vi "Init GU Arrange.vi"(6 "Force Auto(False)":bool, 8 "error in":errorcluster, 9 "Latest Cal Cfg":T1, 10 "Curr Cal Cfg In":T1, 11 "Config Data":T2(array[cluster])) -> (0 "error out":errorcluster, 2 "Curr Cal Cfg Out":T1, 3 "Config Data Out":T2(array[cluster]))   [LabVIEW 2020, in "GUCalibration2.lvlib"]
uses:
  GUCalibration2.lvlib
  Controls/Config Data Type.ctl
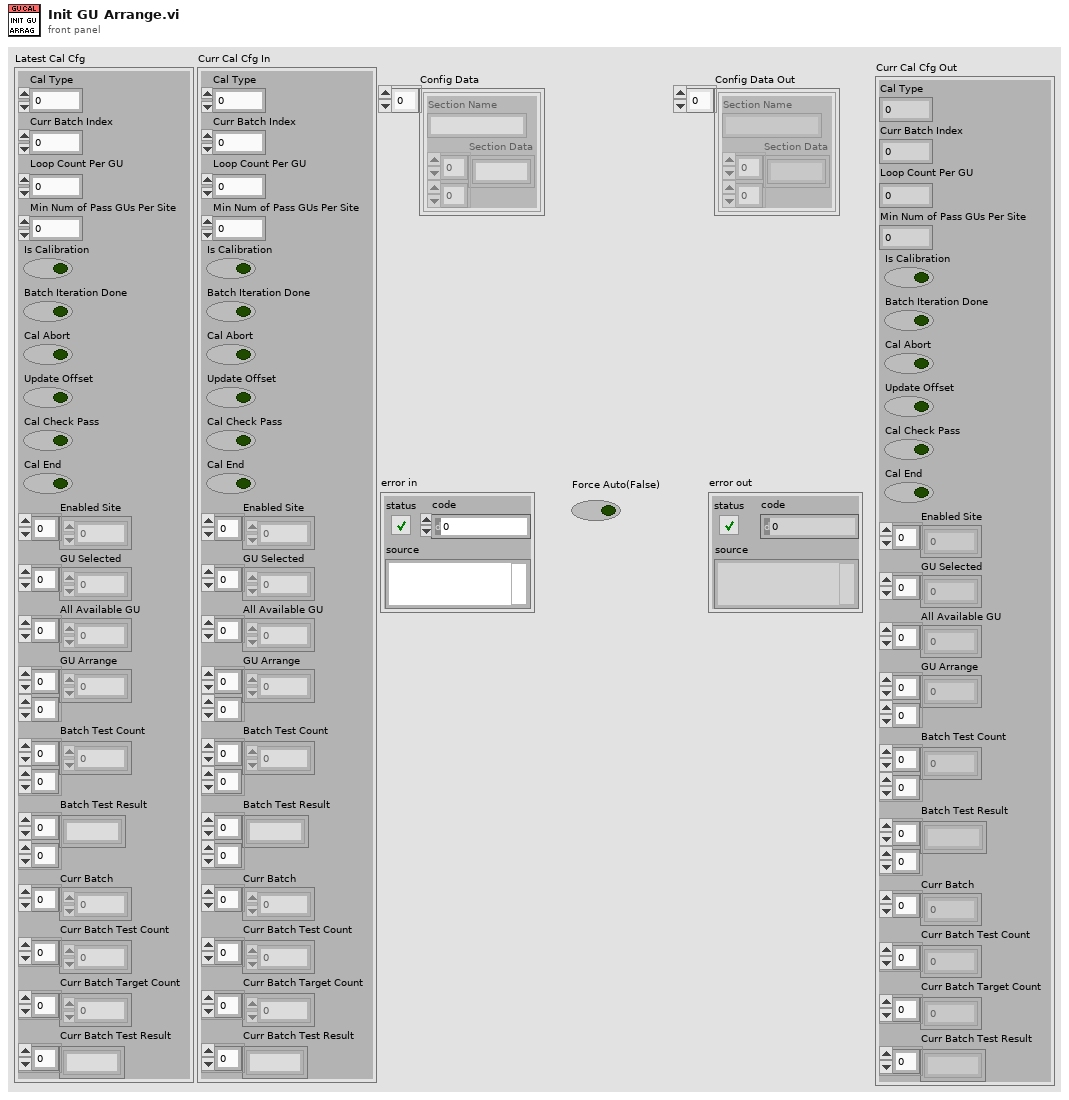
[diagram p1: front panel]
types:
  T1 = typedef "GUCalibration2.lvlib/Config Data Type.ctl" = cluster{"Cal Type":i32, "Curr Batch Index":i32, "Loop Count Per GU":i32, "Min Num of Pass GUs Per Site":i32, "Is Calibration":bool, "Batch Iteration Done":bool, "Cal Abort":bool, "Update Offset":bool, "Cal Check Pass":bool, "Cal End":bool, "Enabled Site":i32[], "GU Selected":i32[], "All Available GU":i32[], "GU Arrange":i32[][], "Batch Test Count":i32[][], "Batch Test Result":string[][], "Curr Batch":i32[], "Curr Batch Test Count":i32[], "Curr Batch Target Count":i32[], "Curr Batch Test Result":string[]}
  T2 = cluster{"Section Name":string, "Section Data":string[][]}[]
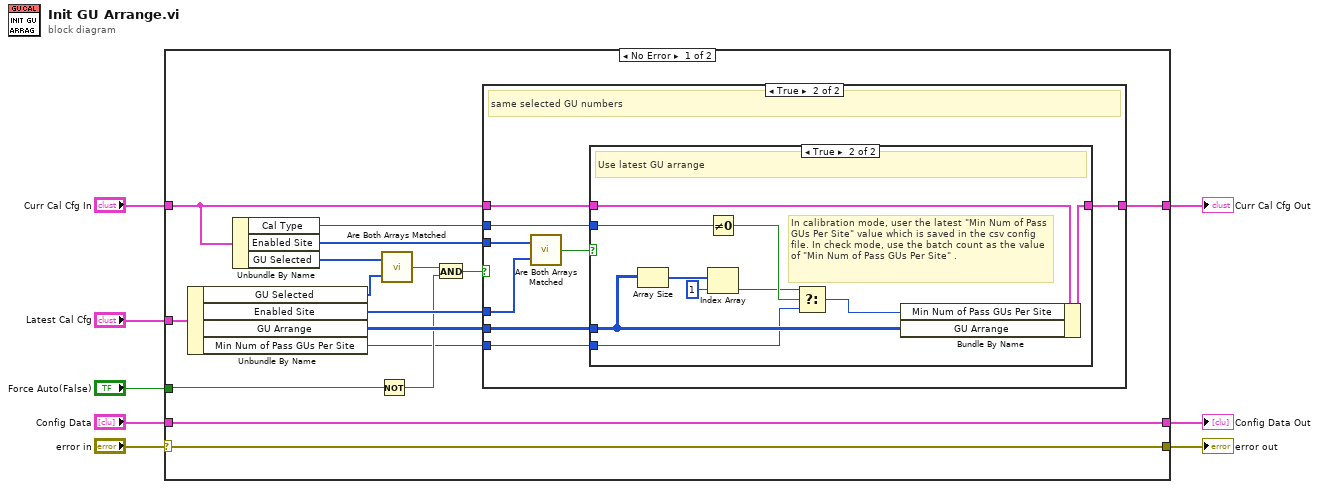
[diagram p0: block diagram]
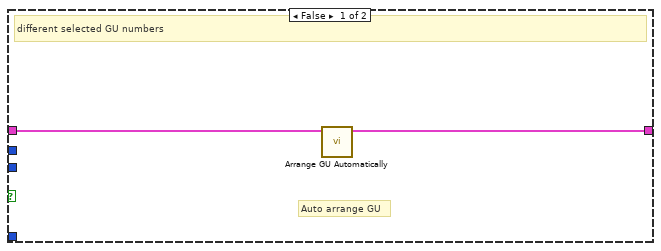
[diagram p2: hidden frame]
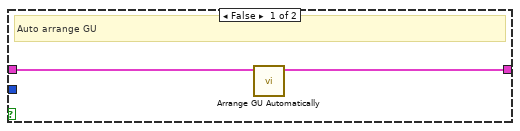
[diagram p3: hidden frame]
diagram:
  n1 = case shown="No Error" "error in" {
    selector: "error in" -> [w16 w49]
    tunnel: [w16 w49] -> w8
    tunnel: "Latest Cal Cfg" -> [w24 _]
    tunnel: "Config Data" -> [w17 w48]
    tunnel: [w17 w48] -> w4
    tunnel: "Curr Cal Cfg In" -> [w19 w47]
    tunnel: [w18 w47] -> w2
    tunnel: "Force Auto(False)" -> [w14 _]
    frame No Error {
      n2 = Unbundle By Name(w24) -> ("GU Selected"=w15:i32[], "Enabled Site"=w22:i32[], "GU Arrange"=w20:i32[][], "Min Num of Pass GUs Per Site"=w10:i32)
      n3 = Unbundle By Name(w19) -> ("Cal Type"=w9:i32, "Enabled Site"=w23:i32[], "GU Selected"=w21:i32[])
      n4 = Not(x=w14) -> (.not. x?=w12:bool)
      n5 = call "Are Both Arrays Matched.vi"("Array2"=w15, "Array1"=w21) -> ("Match ?"=w13:bool)
      n6 = And(x=w13, y=w12) -> (x .and. y?=w11:bool)
      n7 = case shown="True" w11 {
        tunnel: w23 -> [_ w34]
        tunnel: w22 -> [_ w33]
        tunnel: w20 -> [_ w31]
        tunnel: w19 -> [w26 w32]
        tunnel: [w25 w29] -> w18
        tunnel: w10 -> [_ w28]
        tunnel: w9 -> [_ w27]
        frame False {
          # "Auto arrange GU"
          # "different selected GU numbers"
          n8 = call "Arrange GU Automatically.vi"("Curr Cal Cfg In"=w26) -> ("Curr Cal Cfg Out"=w25:T1)  [unwired: 9 in, 1 out]
        }
        frame True {
          # "same selected GU numbers"
          n9 = call "Are Both Arrays Matched.vi"("Array2"=w33, "Array1"=w34) -> ("Match ?"=w30:bool)
          n10 = case shown="True" w30 {
            tunnel: w32 -> [w36 w46]
            tunnel: w31 -> [_ w43]
            tunnel: [w35 w45] -> w29
            tunnel: w28 -> [_ w39]
            tunnel: w27 -> [_ w44]
            frame False {
              # "Auto arrange GU"
              n11 = call "Arrange GU Automatically.vi"("Curr Cal Cfg In"=w36) -> ("Curr Cal Cfg Out"=w35:T1)  [unwired: 9 in, 1 out]
            }
            frame True {
              # "In calibration mode, user the latest \"Min Num of Pass GUs Per Site\" value which is saved in the csv config file. In check mode, use the batch count as the value of \"Min Num of Pass GUs Per Site\" ."
              # "Use latest GU arrange"
              n12 = Array Size(array=w43) -> (size(s)=w42:i32[])
              n13 = Not Equal To 0?(x=w44) -> (x != 0?=w40:bool)
              n14 = Index Array(array=w42, index=1) -> (element=w38:i32)
              n15 = Select(t=w38, s=w40, f=w39) -> (s? t:f=w37:i32)
              n16 = Bundle By Name(cluster=w46, "Min Num of Pass GUs Per Site"=w37, "GU Arrange"=w43) -> (w45:T1)
            }
          }
        }
      }
    }
    frame Error {
    }
  }
  "error out" <- w8
  "Curr Cal Cfg Out" <- w2
  "Config Data Out" <- w4
